vi "SRV_Read More Data.vi"(4 "TCP Settings":T1={"Method"=enum."General", "bytes to read"=65535, "timeout ms (1000)"=10}, 6 "Delay Before Read (10ms)":u32=10, 7 "Read More Data? (T)":bool=TRUE, 8 "error in (no error)":errorcluster, 9 "Data in":string, 11 "Connection ID":refnum<k5>) -> (0 "error out":errorcluster, 1 "Data out":string, 3 "Connection ID out":refnum<k5>)   [LabVIEW 2009]
uses:
  TCP_Communication/SRV_TCP Settings.ctl
  TCP_Communication/SRV_Package Methods.ctl
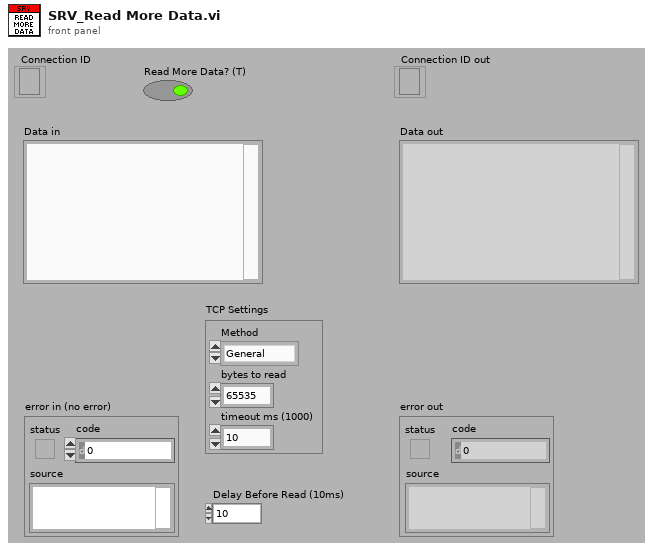
[diagram p1: front panel]
types:
  T1 = typedef "SRV_TCP Settings.ctl" = cluster{"Method":T2, "bytes to read":i32, "timeout ms (1000)":i32}
  T2 = typedef "SRV_Package Methods.ctl" = enum16{"General", "Standard", "CRLF", "Image", "HTML"}
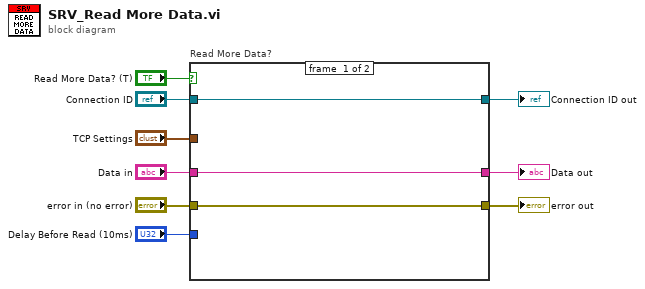
[diagram p0: block diagram]
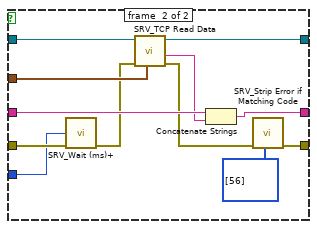
[diagram p2: hidden frame]
diagram:
  n1 = case "Read More Data?" shown="True" "Read More Data? (T)" {
    tunnel: "Connection ID" -> [w11 w18]
    tunnel: [w11 w17] -> w5
    tunnel: "Data in" -> [w12 w23]
    tunnel: [w12 w24] -> w9
    tunnel: "error in (no error)" -> [w10 w15]
    tunnel: [w10 w21] -> w2
    tunnel: "TCP Settings" -> [_ w19]
    tunnel: "Delay Before Read (10ms)" -> [_ w13]
    frame #0 {
    }
    frame #1 {
      n2 = call "SRV_Wait (ms)+.vi"("milliseconds to wait"=w13, "error in (no error)"=w15) -> ("error out"=w14:errorcluster)  [unwired: 12 in, 1 out]
      n3 = call "SRV_TCP Read Data.vi"("TCP Settings"=w19, "error in"=w14, "connection ID in"=w18) -> ("error out"=w20:errorcluster, "data out"=w16:string, "connection ID"=w17:refnum<k5>)  [unwired: 2 in, 1 out]
      n4 = Concatenate Strings(w23, w16) -> (w24:string)
      n5 = call "SRV_Strip Error if Matching Code.vi"("error in (no error)"=w20, "Strip Codes"=i32[] [56]) -> ("error out"=w21:errorcluster)  [unwired: 8 in]
    }
  }
  "Data out" <- w9
  "Connection ID out" <- w5
  "error out" <- w2
